vi "DSP.vi"(5 "err":dbl(knob) scale=-1.2..1.2, 6 "Base":dbl=0.85 step=0.1) -> (1 "Right":dbl, 2 "Left":dbl)   [LabVIEW 2011]
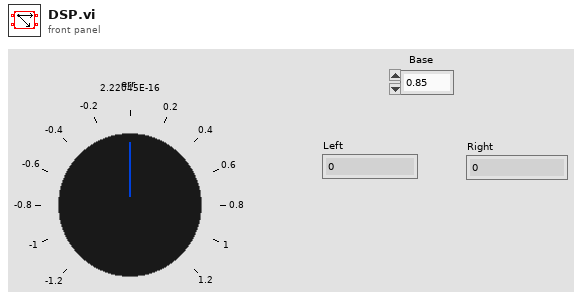
[diagram p1: front panel]
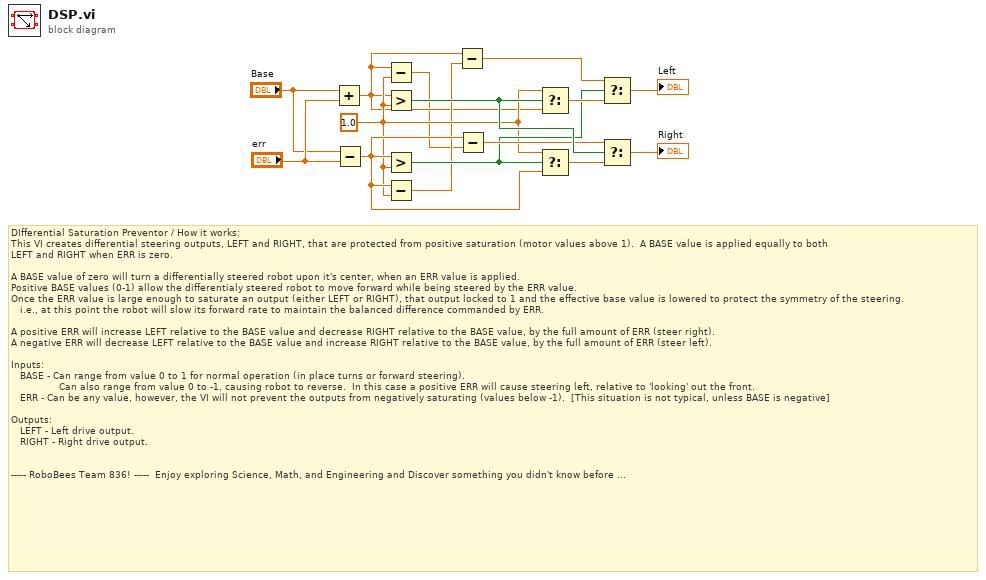
[diagram p0: block diagram]
diagram:
  w4 = 1.0 ("y")
  # "DIfferential Saturation Preventor / How it works:\nThis VI creates differential steering outputs, LEFT and RIGHT, that are protected from positive saturation (motor values above 1).  A BASE value is applied equally to both\nLEFT and RIGHT when ERR is zero.\n\nA BASE value of zero will turn a differentially steered robot upon it's center, when an ERR value is applied.\nPositive BASE values (0-1) allow the differentialy steered robot to move forward while being steered by the ERR value.\nOnce the ERR value is large enough to saturate an output (either LEFT or RIGHT), that output locked to 1 and the effective base value is lowered to protect the symmetry of the steering.\n   i.e., at this point the robot will slow its forward rate to maintain the balanced difference commanded by ERR.\n\nA positive ERR will increase LEFT relative to the BASE value and decrease RIGHT relative to the BASE value, by the full amount of ERR (steer right).\nA negative ERR will decrease LEFT relative to the BASE value and increase RIGHT relative to the BASE value, by the full amount of ERR (steer left).\n\nInputs:\n   BASE - Can range from value 0 to 1 for normal operation (in place turns or forward steering).\n                Can also range from value 0 to -1, causing robot to reverse.  In this case a positive ERR will cause steering left, relative to 'looking' out the front. \n   ERR - Can be any value, however, the VI will not prevent the outputs from negatively saturating (values below -1).  [This situation is not typical, unless BASE is negative]\n\nOutputs:\n   LEFT - Left drive output.\n   RIGHT - Right drive output.\n\n\n----- RoboBees Team 836! -----  Enjoy exploring Science, Math, and Engineering and Discover something you didn't know before ..."
  n1 = Add(x="Base", y="err") -> (x+y=w2:dbl)
  n2 = Subtract(x="Base", y="err") -> (x-y=w5:dbl)
  n3 = Subtract(x=w2, y=w4) -> (x-y=w1:dbl)
  n4 = Greater?(x=w2, y=w4) -> (0:w15:bool)
  n5 = Greater?(x=w5, y=w4) -> (0:w11:bool)
  n6 = Subtract(x=w5, y=w4) -> (x-y=w3:dbl)
  n7 = Subtract(x=w2, y=w3) -> (x-y=w9:dbl)
  n8 = Subtract(x=w5, y=w1) -> (x-y=w13:dbl)
  n9 = Select(t=w4, s=w15, f=w2) -> (s? t:f=w12:dbl)
  n10 = Select(t=w4, s=w11, f=w5) -> (s? t:f=w14:dbl)
  n11 = Select(t=w9, s=w11, f=w12) -> (s? t:f=→"Left":dbl)
  n12 = Select(t=w13, s=w15, f=w14) -> (s? t:f=→"Right":dbl)
